vi "TrackRect.vi"(3 "Debug":bool, 4 "Track":bool, 5 "Mono Image In 2":T4, 6 "Color Image In":T4) -> (0 "Curves":T1[](array[typedef]) {"Points"."Y" format="%.2f"; "Points"."X" format="%.2f"}, 1 "Rects":i32, 2 "ColorImage Out":T4)   [LabVIEW 2017]
uses:
  <vilib>/vision/Image Controls.llb/IMAQ Image.ctl
  <vilib>/vision/Shape Detection.llb/ShapeDetectionMatchOptions.ctl
  <vilib>/vision/Pattern Matching.llb/IMAQ Match Range Setting.ctl
  <vilib>/vision/Pattern Matching.llb/IMAQ Curve Parameters.ctl
  <vilib>/vision/Analysis.llb/IMAQ ExtractCurvesCurve.ctl
  <vilib>/vision/NI_Vision_Development_Module.lvlib
panel:
  out "Rectangles":T2(array[cluster]) {"Corners"."Y" format="%.2f"; "Corners"."X" format="%.2f"}
  in  "Rectangle Descriptor":T3={"Min Width"=10.0, "Max Width"=100.0, "Min Height"=10.0, "Max Height"=100.0}
  in  "Minimum match score":dbl=600.0
  in  "Curve Parameters":T5={"Extraction Mode"=0, "Edge Threshold"=50, "Edge Filter Size"=1, "Min Length"=25, "Row Search Step Size"=15, "Col Search Step Size"=15, "Max Endpoint Gap"=10, "Closed"=FALSE, "Subpixel"=FALSE} {"Extraction Mode" items=["Normal", "Uniform Regions"]; "Edge Filter Size" items=["Fine", "Normal", "Contour Tracing"]; "Max Endpoint Gap" min=0; "Col Search Step Size" min=1 max=255 step=1; "Row Search Step Size" min=1 max=255 step=1; "Min Length" min=0; "Edge Threshold" min=1 max=350 step=1}
  in  "Match Options":T6={"Rotation"=FALSE, "Scale"=FALSE, "Occlusion"=TRUE, "Range Settings"=[{"Match Constraints"=2, "Min"=0.0, "Max"=40.0}]} {"Range Settings"."Max" format="%.2f"; "Range Settings"."Min" format="%.2f"; "Range Settings"."Match Constraints" items=["Rotation Angle (degrees)", "Scale Factor (%)", "Occlusion (%)"]}
  # "Range"
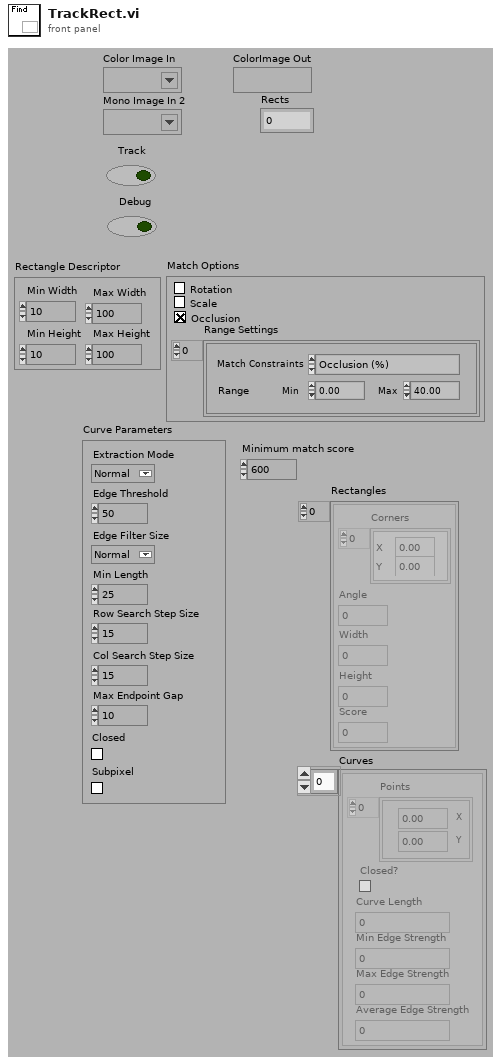
[diagram p1: front panel]
types:
  T1 = typedef "IMAQ ExtractCurvesCurve.ctl" = cluster{"Points":cluster{"X":dbl, "Y":dbl}[], "Closed?":bool, "Curve Length":dbl, "Min Edge Strength":dbl, "Max Edge Strength":dbl, "Average Edge Strength":dbl}
  T2 = cluster{"Corners":cluster{"X":sgl, "Y":sgl}[], "Angle":dbl, "Width":dbl, "Height":dbl, "Score":dbl}[]
  T3 = cluster{"Min Width":dbl, "Max Width":dbl, "Min Height":dbl, "Max Height":dbl}
  T4 = typedef "IMAQ Image.ctl" = refnum<image>
  T5 = typedef "IMAQ Curve Parameters.ctl" = cluster{"Extraction Mode":u32, "Edge Threshold":i32, "Edge Filter Size":u32, "Min Length":i32, "Row Search Step Size":i32, "Col Search Step Size":i32, "Max Endpoint Gap":i32, "Closed":bool, "Subpixel":bool}
  T6 = typedef "ShapeDetectionMatchOptions.ctl" = cluster{"Rotation":bool, "Scale":bool, "Occlusion":bool, "Range Settings":T7[]}
  T7 = typedef "IMAQ Match Range Setting.ctl" = cluster{"Match Constraints":u32, "Min":dbl, "Max":dbl}
  T8 = cluster{"Global Rectangle":i32[], "Contours":cluster{"ID":enum32{"External", "Internal"}, "Type":u32, "Coordinates":i32[]}[]}
  T9 = cluster{"Desired Font (Application)":enum16{"User-specified Font", "Application Font", "System Font", "Dialog Font"}, "[User-specified Font]":cluster{"Font Name":string, "Size":i16, "Strikeout?":bool, "Italic?":bool, "Underline?":bool, "Outline?":bool, "Shadow?":bool, "Bold?":bool, "Rotation Angle":dbl}, "Horizontal Alignment":i16, "Vertical Alignment":i16}
  T10 = typedef "IMAQ Rectangle" = cluster{"Left":i32, "Top":i32, "Right":i32, "Bottom":i32, "Rotation":dbl}
  T11 = typedef "ROI Descriptor" = cluster{"Global Rectangle":i32[], "Contours":cluster{"ID":enum32{"External", "Internal"}, "Type":u32, "Coordinates":i32[]}[]}
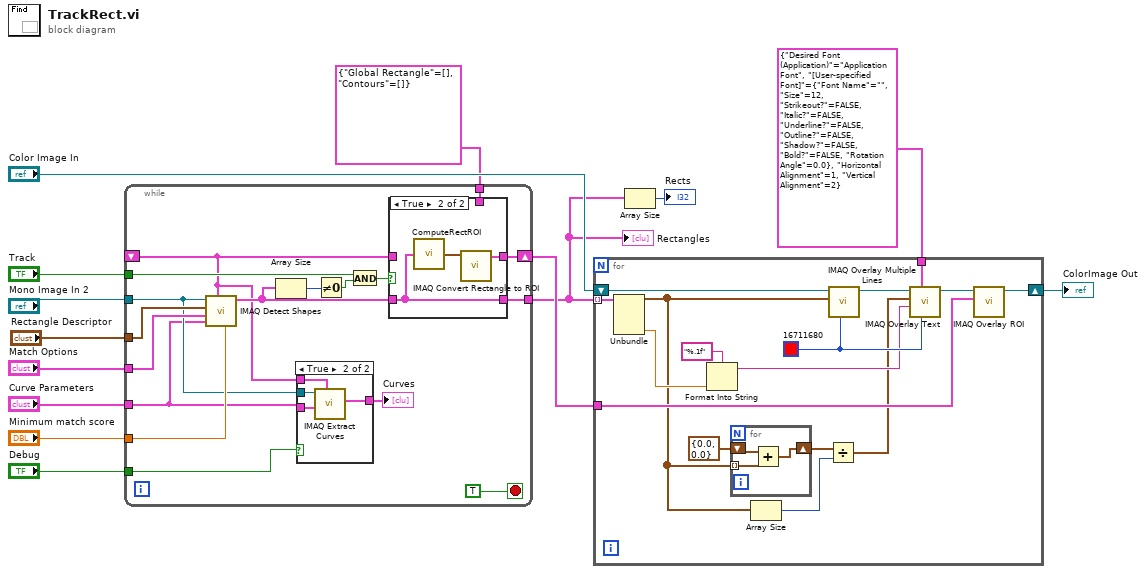
[diagram p0: block diagram]
diagram:
  n1 = while {
    tunnel: [w27] -> w3
    tunnel: "Rectangle Descriptor" -> [w31]
    tunnel: "Match Options" -> [w30]
    tunnel: "Curve Parameters" -> [w16]
    tunnel: "Minimum match score" -> [w29]
    tunnel: "Mono Image In 2" -> [w17]
    shift-right: [w26] -> w5
    shift-left: _ -> [w18]
    tunnel: "Track" -> [w28]
    tunnel: T8 {"Global Rectangle"=[], "Contours"=[]} ("ROI Descriptor") -> [w25]
    tunnel: "Debug" -> [w15]
    stop <- TRUE stop-if-true
    n2 = call-poly "IMAQ Detect Shapes"("Minimum match score"=w29, "Curve Parameters"=w16, "ROI Descriptor"=w18, "Match Options"=w30, "Rectangle Descriptor"=w31, "Image"=w17) -> ("Rectangles"=w22:T2)  [unwired: 3 in, 2 out]
    n3 = Array Size(array=w22) -> (size(s)=w21:i32)
    n4 = case shown="True" w15 {
      tunnel: w16 -> [_ w35]
      tunnel: w17 -> [_ w34]
      tunnel: w18 -> [_ w33]
      tunnel: [_ w32] -> w19
      frame False {
      }
      frame True {
        n5 = call "IMAQ Extract Curves"("ROI Descriptor"=w33, "Curve Parameters"=w35, "Image"=w34) -> ("Curves"=w32:T1[])  [unwired: 6 in, 2 out]
      }
    }
    "Curves" <- w19
    n6 = Not Equal To 0?(x=w21) -> (x != 0?=w20:bool)
    n7 = And(x=w28, y=w20) -> (x .and. y?=w23:bool)
    n8 = case shown="True" w23 {
      tunnel: w18 -> [_ _]
      tunnel: w22 -> [w37 w39]
      tunnel: [w37 w39] -> w27
      tunnel: [w36 w40] -> w26
      tunnel: w25 -> [w36 _]
      frame False {
      }
      frame True {
        n9 = call <vilib>:"ComputeRectROI.vi"("Rectangles"=w39) -> ("Rectangle"=w38:T10)
        n10 = call "IMAQ Convert Rectangle to ROI"("Rectangle"=w38) -> ("ROI Descriptor"=w40:T11)  [unwired: 8 in, 1 out]
      }
    }
  }
  "Rectangles" <- w3
  n11 = for {
    shift-right: [w48] -> w14
    shift-left: "Color Image In" -> [w56]
    tunnel: w3 -> [w55] mode=indexing
    tunnel: T9 {"Desired Font (Application)"=enum."Application Font", "[User-specified Font]"={"Font Name"="", "Size"=12, "Strikeout?"=FALSE, "Italic?"=FALSE, "Underline?"=FALSE, "Outline?"=FALSE, "Shadow?"=FALSE, "Bold?"=FALSE, "Rotation Angle"=0.0}, "Horizontal Alignment"=1, "Vertical Alignment"=2} ("Font, Size & Style") -> [w52]
    tunnel: w5 -> [w47]
    w54 = u32 16711680 ("Color")
    n12 = Unbundle(w55) -> ("Corners"=w43:cluster{"X":sgl, "Y":sgl}[], "Score"=w46:dbl)  [unwired: 3 out]
    n13 = Format Into String(format string="%.1f", w46) -> (resulting string=w51:string)  [unwired: 2 in, 1 out]
    n14 = for {
      tunnel: w43 -> [w59] mode=indexing
      shift-right: [w57] -> w44
      shift-left: cluster{"X":sgl, "Y":sgl} {"X"=0.0, "Y"=0.0} -> [w58]
      n15 = Add(x=w58, y=w59) -> (x+y=w57:cluster{"X":sgl, "Y":sgl})
    }
    n16 = Array Size(array=w43) -> (size(s)=w42:i32)
    n17 = Divide(x=w44, y=w42) -> (x/y=w41:cluster{"X":sgl, "Y":sgl})
    n18 = call "IMAQ Overlay Multiple Lines"("Color"=w54, "Line End Points"=w43, "Image"=w56) -> ("Image Out"=w53:T4)  [unwired: 7 in, 1 out]
    n19 = call "IMAQ Overlay Text"("Text Color (black)"=w54, "Font, Size & Style"=w52, "String"=w51, "Origin"=w41, "Image"=w53) -> ("Image Out"=w49:T4)  [unwired: 5 in, 1 out]
    n20 = call "IMAQ Overlay ROI"("ROI Descriptor"=w47, "Image"=w49) -> ("Image Out"=w48:T4)  [unwired: 8 in, 1 out]
  }
  "ColorImage Out" <- w14
  n21 = Array Size(array=w3) -> (size(s)=→"Rects":i32)
